vi "Post Message To Event Log.vi"(8 "error in (no error)":errorcluster, 9 "Event Type":u16(ring) items=["All", "Error", "Warning", "Informational"], 10 "User Message":string="my Error", 11 "VISA resource name":refnum<visa-resource-name>) -> (0 "error out":errorcluster, 3 "VISA resource name out":refnum<visa-resource-name>)   [LabVIEW 2016, in "Keithley DMM7510.lvlib"]
doc: "This VI allows you to post messages to the event log. You can use this VI to create your own event log entries and assign a severity level to them. This can be useful for debugging and status reporting."
uses:
  Keithley DMM7510.lvlib
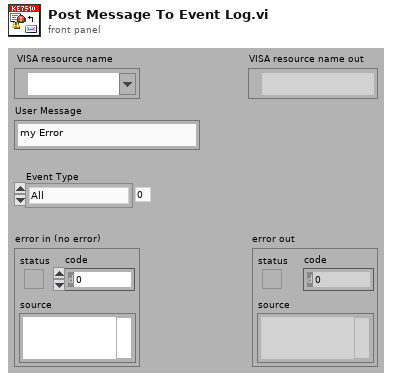
[diagram p1: front panel]
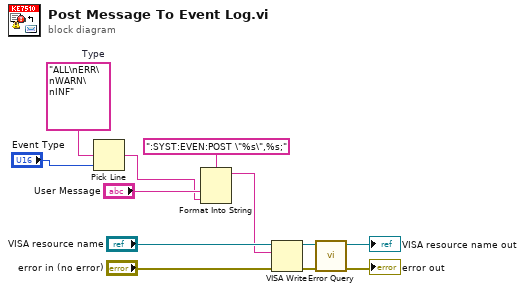
[diagram p0: block diagram]
diagram:
  w2 = "ALL\nERR\nWARN\nINF"  # Type
  n1 = Pick Line(multi-line string=w2, line index="Event Type") -> (output string=w1:string)  [unwired: 1 in]
  n2 = Format Into String(format string=":SYST:EVEN:POST \"%s\",%s;", "User Message", w1) -> (resulting string=w6:string)  [unwired: 2 in, 1 out]
  n3 = VISA Write(VISA resource name="VISA resource name", write buffer=w6, error in (no error)="error in (no error)") -> (VISA resource name out=w8:refnum<visa-resource-name>, error out=w7:errorcluster)  [unwired: 1 out]
  n4 = call "Error Query.vi"("error in (no error)"=w7, "VISA resource name"=w8) -> ("error out"=→"error out":errorcluster, "VISA resource name out"=→"VISA resource name out":refnum<visa-resource-name>)  [unwired: 8 out]
